vi "WPI_SerialPortOpen_USB.vi"(0 "Baud Rate":u32=9600, 1 "Timeout Value (ms)":u32=5000, 2 "Termination Char (0xA = '\\n' = LF)":u8=10 format="%.0x", 3 "Enable Termination Char? (T)":bool=TRUE, 5 "Data Bits":u16=8, 7 "Parity":u16(ring) items=["None", "Odd", "Even", "Mark", "Space"], 9 "Stop Bits":u16(ring)=10 items=["1.0"=10, "1.5"=15, "2.0"=20], 11 "error in (no error)":errorcluster, 12 "Flow Control":u16(ring) items=["None", "XON/XOFF", "RTS/CTS", "XON/XOFF & RTS/CTS", "DTR/DSR", "XON/XOFF & DTR/DSR"], 13 "Serial Port":T1=enum."MXP TTL") -> (4 "SerialPortRef":T2, 15 "error out":errorcluster)   [LabVIEW 2014, in "navX-MXP IMU.lvlib"]
doc: "Opens a reference to the serial port. You must open a reference before using any other VIs on this palette.\n\nThis software is licensed. Open the labview\\readme\\WPI Robotics Library Open Source License.txt file for more information."
uses:
  navX-MXP IMU.lvlib
  <vilib>/Rock Robotics/WPI/SerialPort/WPI_SerialPortRef.ctl
  WPI_SerialPort_USB.ctl
  <vilib>/Rock Robotics/SystemInterfaces/NetworkCommunication/NetComm_UsageReport_ResourceType.ctl
panel:
  out "Instrument Name":string
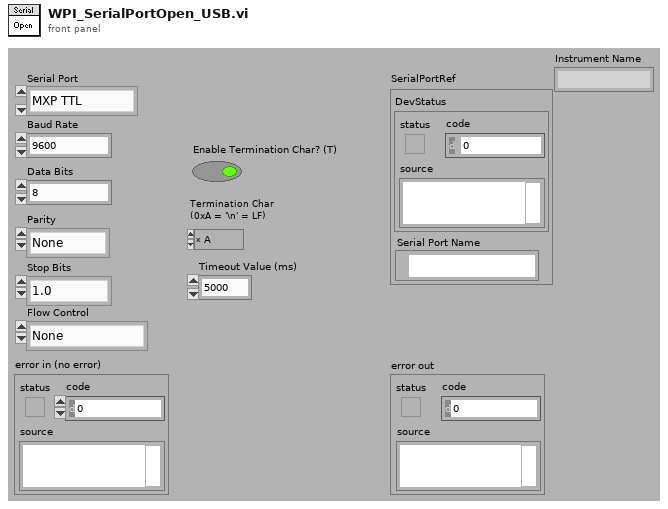
[diagram p1: front panel]
types:
  T1 = typedef "navX-MXP IMU.lvlib/WPI_SerialPort_USB.ctl" = enum16{"Onboard RS-232", "MXP TTL", "USB"}
  T2 = typedef "WPI_SerialPortRef.ctl" = cluster{"DevStatus":errorcluster, "Serial Port Name":refnum<visa-resource-name>}
  T3 = typedef "NetComm_UsageReport_ResourceType.ctl" = enum8{"Controller", "Module", "Language", "CANPlugin", "Accelerometer", "ADXL345", "AnalogChannel", "AnalogTrigger", "AnalogTriggerOutput", "CANJaguar", "Compressor", "Counter", "Dashboard", "DigitalInput", "DigitalOutput", "DriverStationCIO", "DriverStationEIO", "DriverStationLCD", "Encoder", "GearTooth", "Gyro", "I2C", "Framework", "Jaguar", "Joystick", "Kinect", "KinectStick", "PIDController", "Preferences", "PWM", "Relay", "RobotDrive", "SerialPort", "Servo", "Solenoid", "SPI", "Task", "Ultrasonic", "Victor", "Button", "Command", "AxisCamera", "PCVideoServer", "SmartDashboard", "Talon", "HiTechnicColorSensor", "HiTechnicAccel", "HiTechnicCompass", "SRF08", "AnalogOutput", "Victor SP", "Talon SRX", "CAN Talon SRX"}
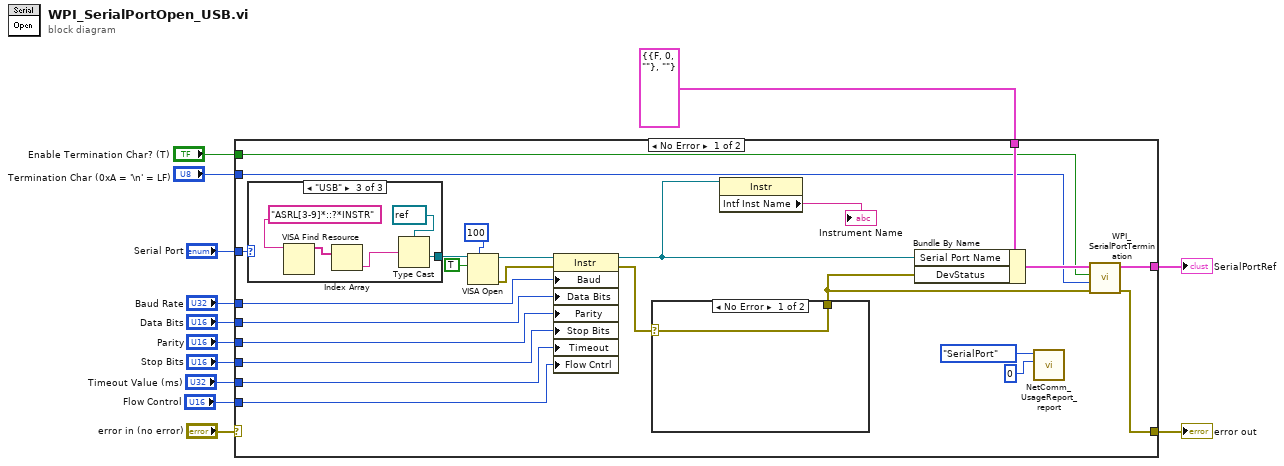
[diagram p0: block diagram]
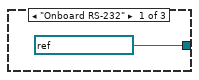
[diagram p2: hidden frame]
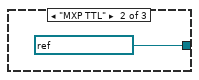
[diagram p3: hidden frame]
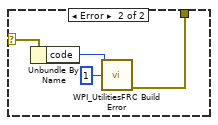
[diagram p4: hidden frame]
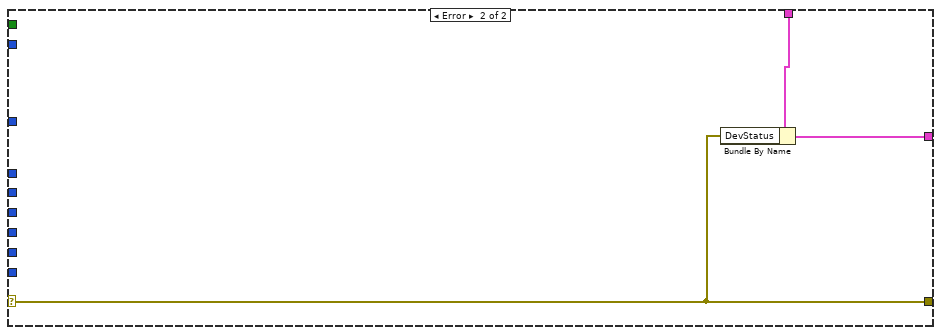
[diagram p5: hidden frame]
diagram:
  n1 = case shown="No Error" "error in (no error)" {
    selector: "error in (no error)" -> [_ w51]
    tunnel: "Baud Rate" -> [w35 _]
    tunnel: "Parity" -> [w34 _]
    tunnel: "Data Bits" -> [w33 _]
    tunnel: [w28 w52] -> w10
    tunnel: "Stop Bits" -> [w24 _]
    tunnel: [w29 w51] -> w7
    tunnel: T2 {"DevStatus"={"status"=FALSE, "code"=0, "source"=""}, "Serial Port Name"=""} ("SerialPortRef") -> [w32 w50]
    tunnel: "Enable Termination Char? (T)" -> [w26 _]
    tunnel: "Termination Char (0xA = '\\n' = LF)" -> [w27 _]
    tunnel: "Timeout Value (ms)" -> [w25 _]
    tunnel: "Flow Control" -> [w23 _]
    tunnel: "Serial Port" -> [w18 _]
    frame No Error {
      n2 = case shown="\"USB\"" w18 {
        tunnel: [refnum<visa-resource-name> "ASRL1::INSTR" ("VISA resource name") refnum<visa-resource-name> "ASRL2::INSTR" ("VISA resource name") w40] -> w17
        frame "Onboard RS-232" {
        }
        frame "MXP TTL" {
        }
        frame "USB" {
          n3 = VISA Find Resource(11:"ASRL[3-9]*::?*INSTR") -> (3:w44:string[])  [unwired: 2 in, 2 out]
          n4 = Index Array(array=w44) -> (element=w42:string)  [unwired: 1 in]
          n5 = Type Cast(type=refnum<visa-resource-name> refnum ("VISA resource name"), x=w42) -> (*(type *) &x=w40:refnum<visa-resource-name>)
        }
      }
      n6 = VISA Open(timeout (0)=100, duplicate session (F)=TRUE, VISA resource name=w17) -> (VISA resource name=w37:refnum<visa-resource-name>, error out=w36:errorcluster)  [unwired: 1 in, 1 out]
      n7 = property class="Instr"(reference=w37, error in=w36, "Baud"=w35, "Data Bits"=w33, "Parity"=w34, "Stop Bits"=w24, "Timeout"=w25, "Flow Cntrl"=w23) -> (reference out=w16:refnum<visa-resource-name>, error out=w22:errorcluster)
      n8 = case shown="No Error" w22 {
        selector: w22 -> [w45 w47]
        tunnel: [w45 w46] -> w21
        frame No Error {
        }
        frame Error {
          n9 = Unbundle By Name(w47) -> ("code"=w49:i32)
          n10 = call <vilib>:"WPI_UtilitiesFRC Build Error.vi"("error code"=w49, "chain levels to remove (1)"=1) -> ("error out"=w46:errorcluster)  [unwired: 3 in, 10 out]
        }
      }
      n11 = property class="Instr"(reference=w16) -> ("Intf Inst Name"=→"Instrument Name":string)  [unwired: 1 in, 2 out]
      n12 = Bundle By Name(cluster=w32, "Serial Port Name"=w16, "DevStatus"=w21) -> (w30:T2)
      n13 = call <vilib>:"NetComm_UsageReport_report.vi"("Instance Number"=u8 0, "Resource Type"=NetComm_UsageReport_ResourceType."SerialPort") -> ()  [unwired: 10 in]
      n14 = call <vilib>:"WPI_SerialPortTermination.vi"("error in (no error)"=w21, "Termination Char (0xA = '\\n' = LF)"=w27, "Enable? (T)"=w26, "SerialPortRef"=w30) -> ("error out"=w29:errorcluster, "SerialPortRef"=w28:T2)  [unwired: 6 out]
    }
    frame Error {
      n15 = Bundle By Name(cluster=w50, "DevStatus"=w51) -> (w52:T2)
    }
  }
  "error out" <- w7
  "SerialPortRef" <- w10
